vi "5p1_HW_Task1B_doanbs.vi"() -> ()   [LabVIEW 2016]
uses:
  <vilib>/express/express arith-compare/Formula/XNode/ExpressFormulaBlockNode.xnode
panel:
  out "S, Stopping Sight Distance (ft)":dbl
  in  "Uphill or Downhill":string(combo)
  in  "tr, Reaction Time (s)":dbl
  in  "G, % Grade divided by 100":dbl
  in  "f, Coefficient of Friction":dbl
  in  "V, Vehicle Speed (mph)":dbl
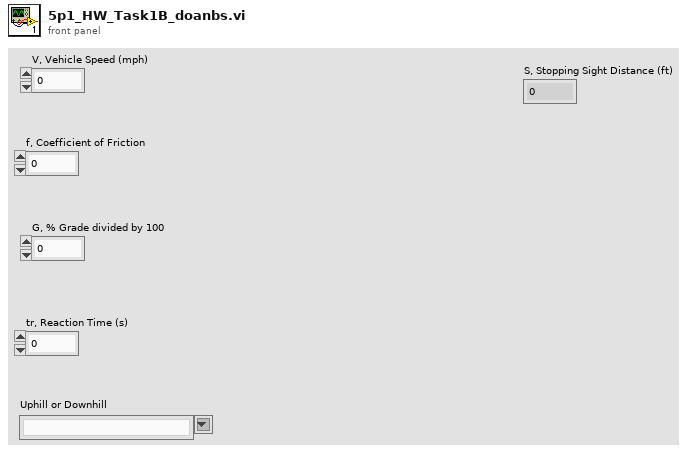
[diagram p1: front panel]
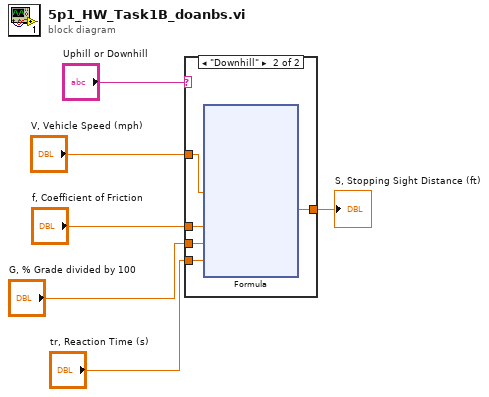
[diagram p0: block diagram]
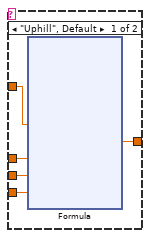
[diagram p2: hidden frame]
diagram:
  n1 = case shown="\"Downhill\"" "Uphill or Downhill" {
    tunnel: "V, Vehicle Speed (mph)" -> [w11 w30]
    tunnel: "f, Coefficient of Friction" -> [w10 w29]
    tunnel: "G, % Grade divided by 100" -> [w9 w28]
    tunnel: "tr, Reaction Time (s)" -> [w8 w27]
    tunnel: [w7 w26] -> w1
    frame "Uphill", Default {
      n2 = xnode "Formula"("V"=w11, "f"=w10, "G"=w9, "tr"=w8) -> ("Result"=w7:dbl)  [unwired: 1 in, 1 out]
    }
    frame "Downhill" {
      n3 = xnode "Formula"("V"=w30, "f"=w29, "G"=w28, "tr"=w27) -> ("Result"=w26:dbl)  [unwired: 1 in, 1 out]
    }
  }
  "S, Stopping Sight Distance (ft)" <- w1
